vi "Global 1.vi"() -> ()   [LabVIEW 2023]
panel:
  in  "Array":void[](array[numeric])
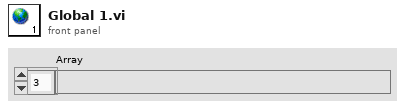
[diagram p1: front panel]
diagram:
